vi "set_params.vi"(8 "error in (no error)":errorcluster, 11 "dummy in":refnum<class "dummy.lvclass">) -> (0 "error out":errorcluster, 3 "dummy out":refnum<class "dummy.lvclass">)   [LabVIEW 2019, in "dummy.lvlib" / "dummy.lvclass"]
uses:
  dummy.lvclass
  C:/Users/lars/Desktop/TransientAbsorptionDAQ/_camera/_camera.lvlibp/_cameraClass/_camera.lvclass
  _camera/_camera.lvlibp/_cameraClass/Write camera name and version.vi
  _camera/_camera.lvlibp/_cameraClass/Write wavelength.vi
panel:
  in  "OK Button":bool
  in  "max":dbl=750.0
  in  "min":dbl=350.0
  # "set wavelength range"
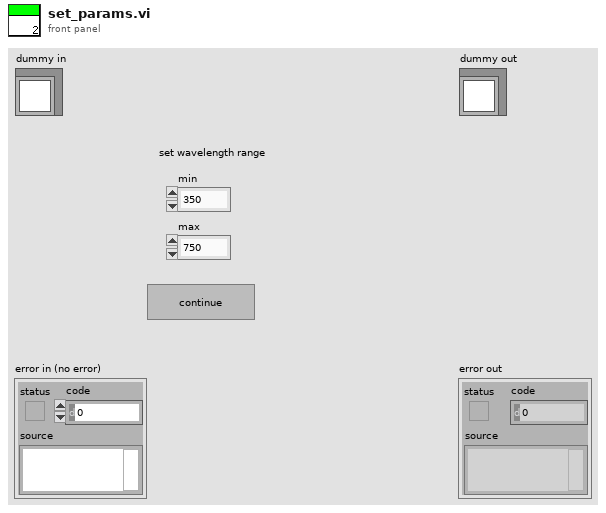
[diagram p1: front panel]
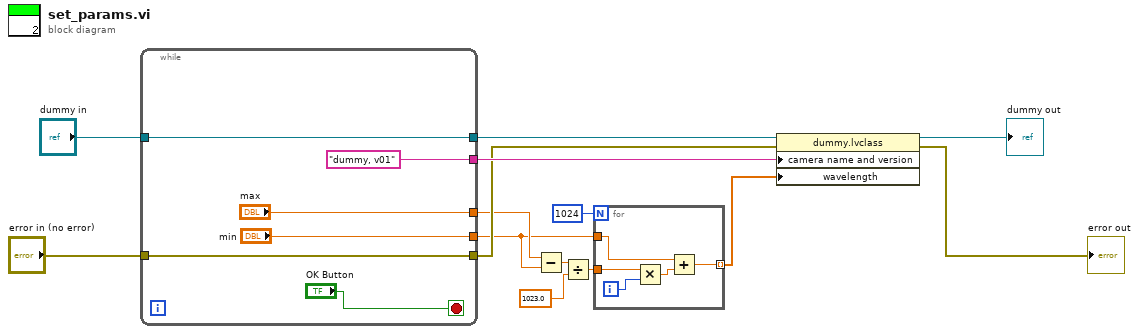
[diagram p0: block diagram]
diagram:
  n1 = while {
    tunnel: "error in (no error)" -> [w20]
    tunnel: [w20] -> w9
    tunnel: "dummy in" -> [w19]
    tunnel: [w19] -> w12
    tunnel: ["dummy, v01" ("camera name, version")] -> w10
    tunnel: ["max"] -> w6
    tunnel: ["min"] -> w5
    stop <- "OK Button" stop-if-true
  }
  n2 = Subtract(x=w6, y=w5) -> (x-y=w4:dbl)
  n3 = Divide(x=w4, y=1023.0) -> (x/y=w2:dbl)
  n4 = for {
    N: 1024 -> [_]
    tunnel: w5 -> [w22]
    tunnel: w2 -> [w25]
    tunnel: [w21] -> w1 mode=indexing
    i -> [w24]
    n5 = Multiply(x=w25, y=w24) -> (x*y=w23:dbl)
    n6 = Add(x=w22, y=w23) -> (x+y=w21:dbl)
  }
  n7 = property class="dummy.lvclass"(reference=w12, error in=w9, "camera name and version"=w10, "wavelength"=w1) -> (reference out=→"dummy out":refnum<class "dummy.lvclass">, error out=→"error out":errorcluster)
